vi "MOKE_Teperature and FIeld Sweep_1022D.vi"() -> ()   [LabVIEW 2022 SP3]
uses:
  <vilib>/Analysis/baseanly.llb/Mean (DBL).vi
  <vilib>/Utility/file.llb/Write Delimited Spreadsheet (string).vi
  <vilib>/Utility/file.llb/Write Delimited Spreadsheet (DBL).vi
  <vilib>/Analysis/NI_AALBase.lvlib
panel:
  in  "Num Averages":i32=100
  in  "Read Status":bool
  in  "Wait for position/focus check every (Oe)":i32
  out "Rh1 B/A v F":cluster{dbl[], dbl[]}(graph)
  out "Temperature Status":i32(ring) items=["TemperatureUnknown"=0, "Stable"=1, "Tracking"=2, "Near"=5, "Chasing"=6, "Filling"=7, "Standby"=10, "Disabled"=13, "ImpedanceNotFunction"=14, "TempFailure"=15]
  out "Field Status":i32(ring) items=["MagnetUnknown"=0, "StablePersistent"=1, "WarmingSwitch"=2, "CoolingSwitch"=3, "StableDriven"=4, "Iterating"=5, "Charging"=6, "Discharging"=7, "CurrentError"=8, "MagnetFailure"=15]
  out "Field":dbl
  out "Temperature":dbl
  in  "Initialize":bool
  in  "System Stablization (s)":dbl=0.1 format="%#_13g"
  in  "Low Value (Oe)":dbl=-30000.0
  in  "High Value (Oe)":dbl=30000.0
  in  "Sweep Field Approach":i32(ring) items=["Linear", "NoOvershoot", "Oscillate"]
  in  "Sweep F Rate (Oe/s)":dbl=200.0 format="%#_13g"
  in  "Sweep F mode":i32(ring) items=["Persistent", "Driven"]
  in  "Set Fixed T":dbl=2.0
  in  "Fixed Temperature Approach":i32(ring)=1 items=["FastSettle", "NoOvershoot"]
  in  "FIxed T  Rate (K/min)":dbl=20.0
  out "PhaseA-F":cluster{dbl[], dbl[]}(graph)
  out "RA-F":cluster{dbl[], dbl[]}(graph)
  out "Phaseh1B-F":cluster{dbl[], dbl[]}(graph)
  out "Rh1B-F":cluster{dbl[], dbl[]}(graph)
  out "phase B 2":dbl
  in  "Phase B 2":u16(ring)=3 items=["X", "Y", "R", "Theta", "Frequency", "Noise", "Xh1", "Yh1", "Rh1", "Theta h1", "Xh2", "Yh2", "Rh2", "Theta h2"]
  out "phase A 2":dbl
  in  "Phase A 2":u16(ring)=3 items=["X", "Y", "R", "Theta", "Frequency", "Noise", "Xh1", "Yh1", "Rh1", "Theta h1", "Xh2", "Yh2", "Rh2", "Theta h2"]
  out "para1 Measurement (mV) 2":dbl=1.49013e-07
  in  "F Clear Plot A":bool
  in  "Parameter A 2":u16(ring)=2 items=["X", "Y", "R", "Theta", "Frequency", "Noise", "Xh1", "Yh1", "Rh1", "Theta h1", "Xh2", "Yh2", "Rh2", "Theta h2"]
  out "para2 Measurement (uV) 2":dbl=1.49013e-07
  in  "F Clear Plot B":bool
  in  "Parameter B 2":u16(ring)=2 items=["X", "Y", "R", "Theta", "Frequency", "Noise", "Xh1", "Yh1", "Rh1", "Theta h1", "Xh2", "Yh2", "Rh2", "Theta h2"]
  out "Field Setting":dbl format="%#_13g"
  out "Fixed Temperature":dbl
  out "Measured Field":dbl
  out "Field Status":i32(ring) items=["MagnetUnknown"=0, "StablePersistent"=1, "WarmingSwitch"=2, "CoolingSwitch"=3, "StableDriven"=4, "Iterating"=5, "Charging"=6, "Discharging"=7, "CurrentError"=8, "MagnetFailure"=15]
  out "Temperature Status":i32(ring) items=["TemperatureUnknown"=0, "Stable"=1, "Tracking"=2, "Near"=5, "Chasing"=6, "Filling"=7, "Standby"=10, "Disabled"=13, "ImpedanceNotFunction"=14, "TempFailure"=15]
  out "Measuring F":bool
  in  "Step(Oe)":i32=2000
  out "F loop run":i32
  out "Temperature Status":i32(ring) items=["TemperatureUnknown"=0, "Stable"=1, "Tracking"=2, "Near"=5, "Chasing"=6, "Filling"=7, "Standby"=10, "Disabled"=13, "ImpedanceNotFunction"=14, "TempFailure"=15]
  out "Field Status":i32(ring) items=["MagnetUnknown"=0, "StablePersistent"=1, "WarmingSwitch"=2, "CoolingSwitch"=3, "StableDriven"=4, "Iterating"=5, "Charging"=6, "Discharging"=7, "CurrentError"=8, "MagnetFailure"=15]
  out "Fixed Field":dbl
  out "Measured Temperature":dbl
  in  "Delay(T/F)":dbl=5.0
  in  "Set FIxed F (Oe)":dbl format="%#_13g"
  in  "Fixed Field Approach":i32(ring) items=["Linear", "NoOvershoot", "Oscillate"]
  in  "FIxed F Rate (Oe/s)":dbl=100.0 format="%#_13g"
  in  "Fixed F mode":i32(ring) items=["Persistent", "Driven"]
  in  "Sweep Temperature Approach":i32(ring)=1 items=["FastSettle", "NoOvershoot"]
  in  "Sweep T  Rate (K/min)":dbl=10.0
  in  "Sweep T/F":bool
  in  "Remote":bool=TRUE
  in  "IP Address":string="169.254.170.239"
  out "Measuring T":bool
  in  "A Sine Output Amplitude (V)":sgl=0.1
  in  "path (folder + filename)":string="C:\\Users\\Public\\OneDrive\\Desktop\\MOKE program\\sweep files"
  in  "LOCKIN address":refnum<visa-resource-name>="COM3"
  out "PhaseA-T":cluster{dbl[], dbl[]}(graph)
  out "RA-T":cluster{dbl[], dbl[]}(graph)
  out "Phaseh1-T":cluster{dbl[], dbl[]}(graph)
  out "Rh1B-T":cluster{dbl[], dbl[]}(graph)
  out "phase B":dbl
  in  "Phase B":u16(ring)=9 items=["X", "Y", "R", "Theta", "Frequency", "Noise", "Xh1", "Yh1", "Rh1", "Theta h1", "Xh2", "Yh2", "Rh2", "Theta h2"]
  out "phase A":dbl
  in  "Phase A":u16(ring)=3 items=["X", "Y", "R", "Theta", "Frequency", "Noise", "Xh1", "Yh1", "Rh1", "Theta h1", "Xh2", "Yh2", "Rh2", "Theta h2"]
  out "para1 Measurement (mV)":dbl=1.49013e-07
  in  "T Clear Plot A":bool
  in  "Parameter A":u16(ring)=2 items=["X", "Y", "R", "Theta", "Frequency", "Noise", "Xh1", "Yh1", "Rh1", "Theta h1", "Xh2", "Yh2", "Rh2", "Theta h2"]
  out "para2 Measurement (uV)":dbl=1.49013e-07
  in  "T Clear Plot B":bool
  in  "Parameter B":u16(ring)=8 items=["X", "Y", "R", "Theta", "Frequency", "Noise", "Xh1", "Yh1", "Rh1", "Theta h1", "Xh2", "Yh2", "Rh2", "Theta h2"]
  out "Temperature Setting":dbl format="%#_13g"
  in  "Save data or not":bool=TRUE
  in  "Step(K)":i32=10
  out "T loop run":i32
  in  "B frequency":dbl=267.7 format="%#_13g"
  in  "B Input Connection (0: Single-Ended)":u16(ring)=1 items=["Single-Ended Voltage", "Differential Voltage", "1 MOhm Current Gain", "100 MOhm Current Gain"]
  in  "B harmonic 1":u8=2
  in  "B harmonic 2":u8=3
  in  "B reference Manual Phase":dbl=-59.75
  in  "auto phase B":bool=TRUE
  in  "B Sample time (s)":dbl=0.001 min=0.001 max=100.0 step=0.001
  in  "B Sensitivity":u16(ring)=20 items=["1 nV/fA", "2 nV/fA", "5 nV/fA", "10 nV/fA", "20 nV/fA", "50 nV/fA", "100 nV/fA", "200 nV/fA", "500 nV/fA", "1 uV/pA", "2 uV/pA", "5 uV/pA", "10 uV/pA", "20 uV/pA", "50 uV/pA", "100 uV/pA", "200 uV/pA", "500 uV/pA", "1 mV/nA", "2 mV/nA", "5 mV/nA", "10 mV/nA", "20 mV/nA", "50 mV/nA", "100 mV/nA", "200 mV/nA", "500 mV/nA", "1 V/uA"]
  in  "Enable Sync Filter B (open when f<200Hz)":bool
  in  "B Time Constant":u8(ring)=9 items=["10 us", "30 us", "100 us", "300 us", "1 ms", "3 ms", "10 ms", "30 ms", "100 ms", "300 ms", "1 s", "3 s", "10 s", "30 s", "100 s", "300 s", "1 ks", "3 ks"]
  in  "B Reference Source":u8(ring) items=["External", "Internal", "Internal Sweep", "Channel-A"]
  in  "B Low Pass Filter Slope":u8(ring)=2 items=["6 dB/oct", "12 dB/oct", "18 db/oct", "24 dB/oct"]
  in  "A frequency":dbl=267.7 format="%#_13g"
  in  "A Input Connection (0: Single-Ended)":u16(ring)=1 items=["Single-Ended Voltage", "Differential Voltage", "1 MOhm Current Gain", "100 MOhm Current Gain"]
  in  "A harmonic 1":u8=2
  in  "A harmonic 2":u8=3
  in  "A reference Manual Phase":dbl=-59.75
  in  "auto phase A":bool=TRUE
  in  "A Reference Source":u8(ring)=1 items=["External", "Internal", "Internal Sweep"]
  in  "A Sample time (s)":dbl=0.001 min=0.001 max=100.0 step=0.001
  in  "A Time Constant":u8(ring)=9 items=["10 us", "30 us", "100 us", "300 us", "1 ms", "3 ms", "10 ms", "30 ms", "100 ms", "300 ms", "1 s", "3 s", "10 s", "30 s", "100 s", "300 s", "1 ks", "3 ks"]
  in  "Enable Sync Filter A (open when f<200Hz)":bool
  in  "A Sensitivity":u16(ring)=20 items=["1 nV/fA", "2 nV/fA", "5 nV/fA", "10 nV/fA", "20 nV/fA", "50 nV/fA", "100 nV/fA", "200 nV/fA", "500 nV/fA", "1 uV/pA", "2 uV/pA", "5 uV/pA", "10 uV/pA", "20 uV/pA", "50 uV/pA", "100 uV/pA", "200 uV/pA", "500 uV/pA", "1 mV/nA", "2 mV/nA", "5 mV/nA", "10 mV/nA", "20 mV/nA", "50 mV/nA", "100 mV/nA", "200 mV/nA", "500 mV/nA", "1 V/uA"]
  in  "A Low Pass Filter Slope":u8(ring)=2 items=["6 dB/oct", "12 dB/oct", "18 db/oct", "24 dB/oct"]
  in  "stabilization(S)":dbl=0.1 format="%#_13g"
  in  "High Value (K)":dbl=300.0
  in  "Low Value (K)":dbl=2.0
  in  "loop #":i32=1
  # "Status"
  # "opticool ip addresse: 169.254.170.239"
  # "Lock-in Setting"
  # "Channel A"
  # "Channel B"
  # "Sweep F Mesurement"
  # "Temprature and Field Setting"
  # "Sweep T Mesurement"
  # "Sweep F"
  # "Sweep T"
  # "0 for no checks"
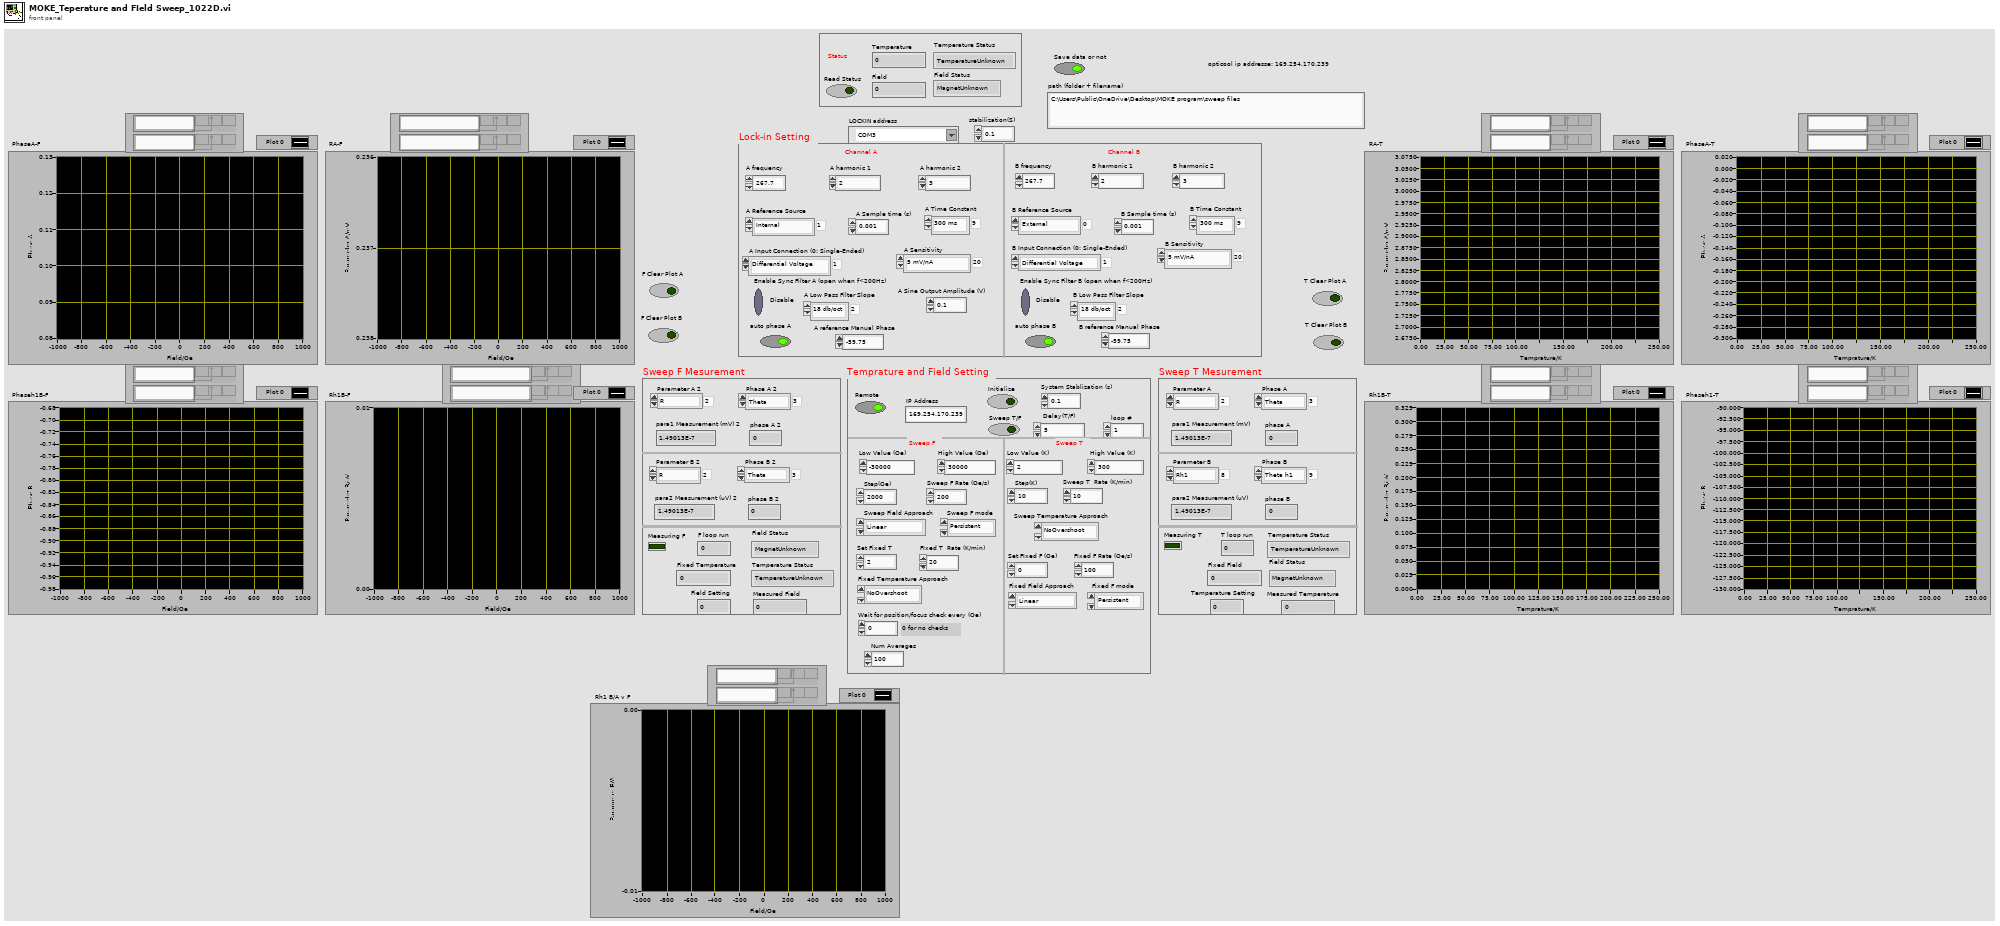
[diagram p1: front panel]
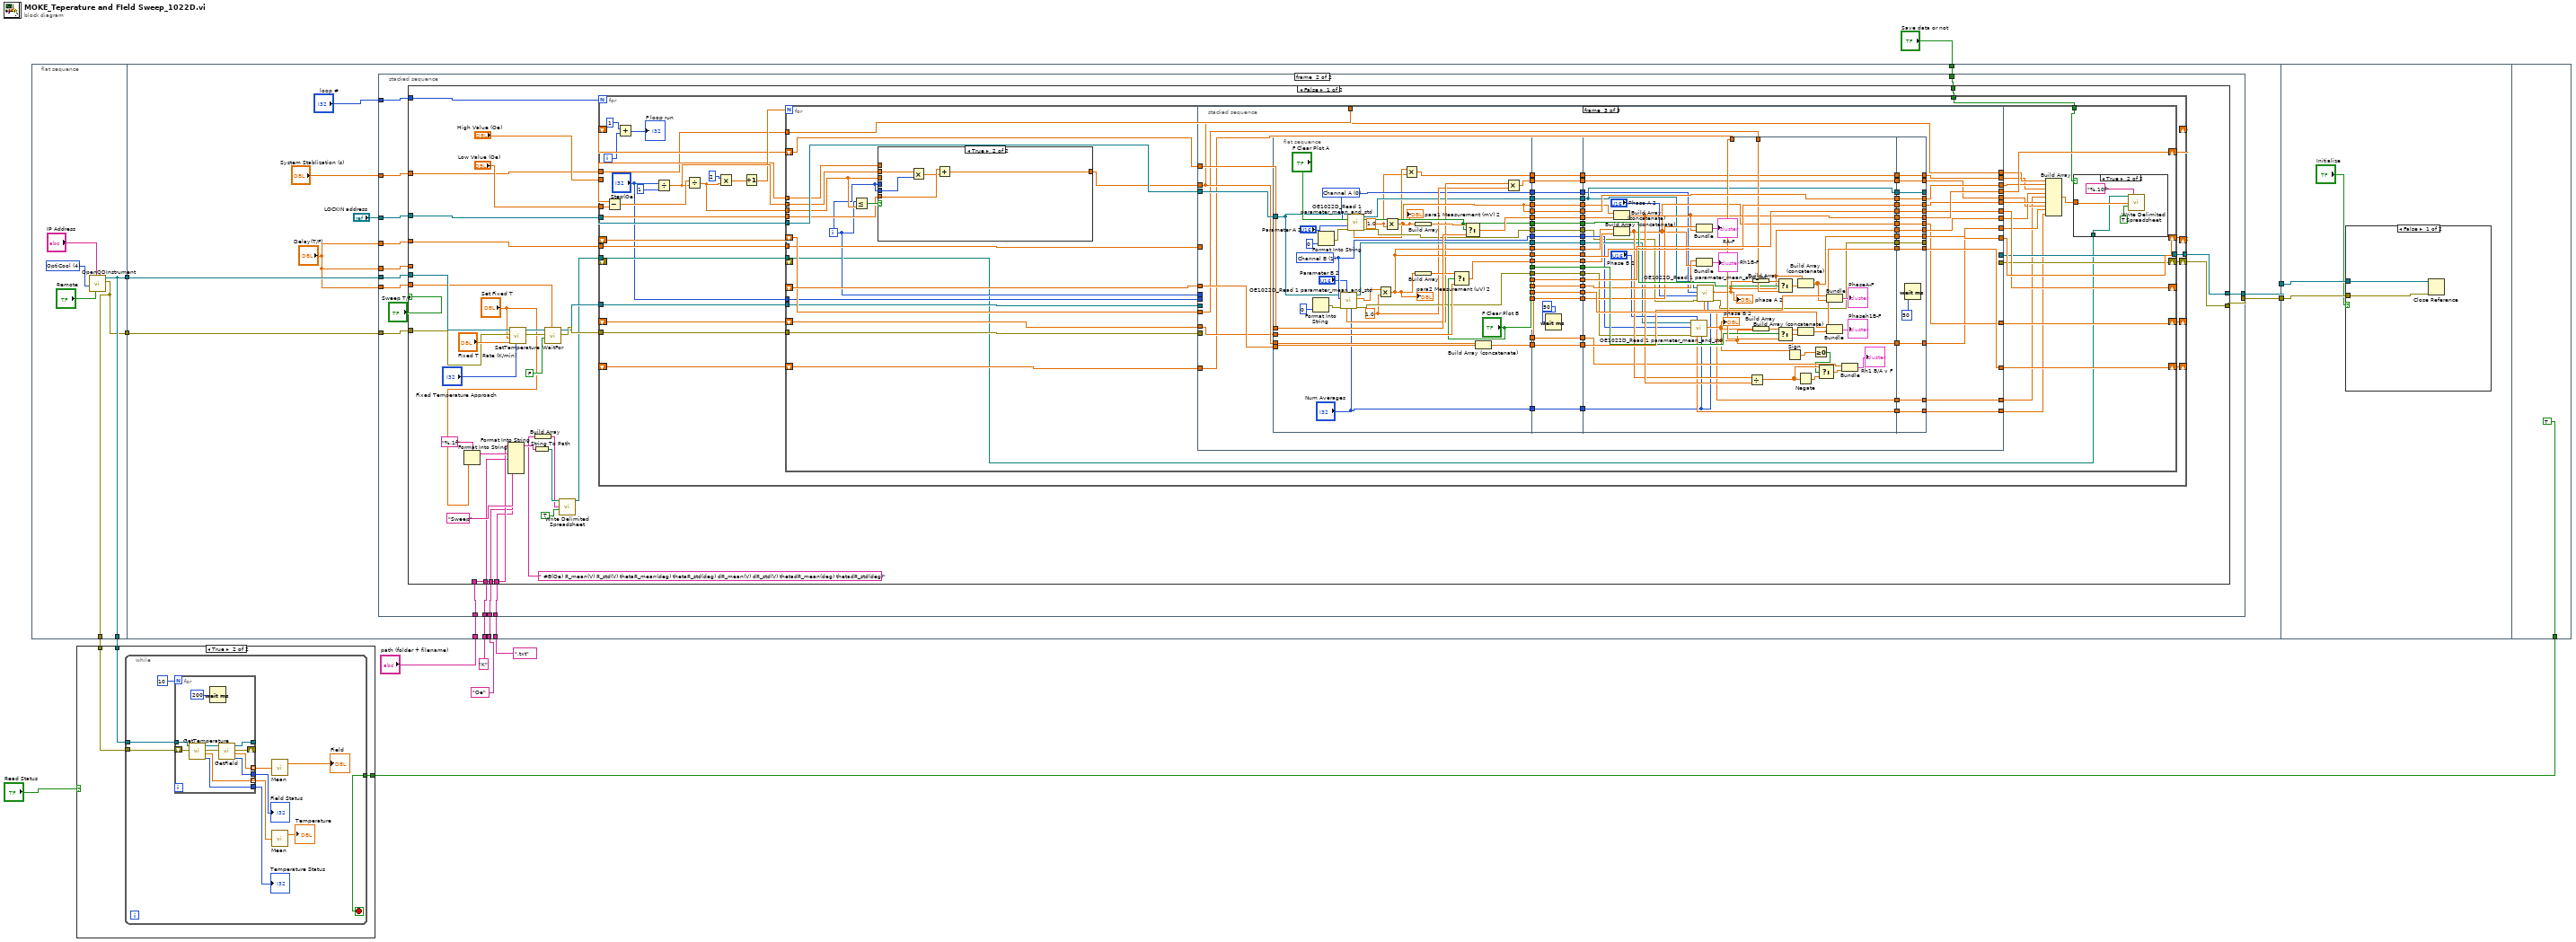
[diagram p0: block diagram]
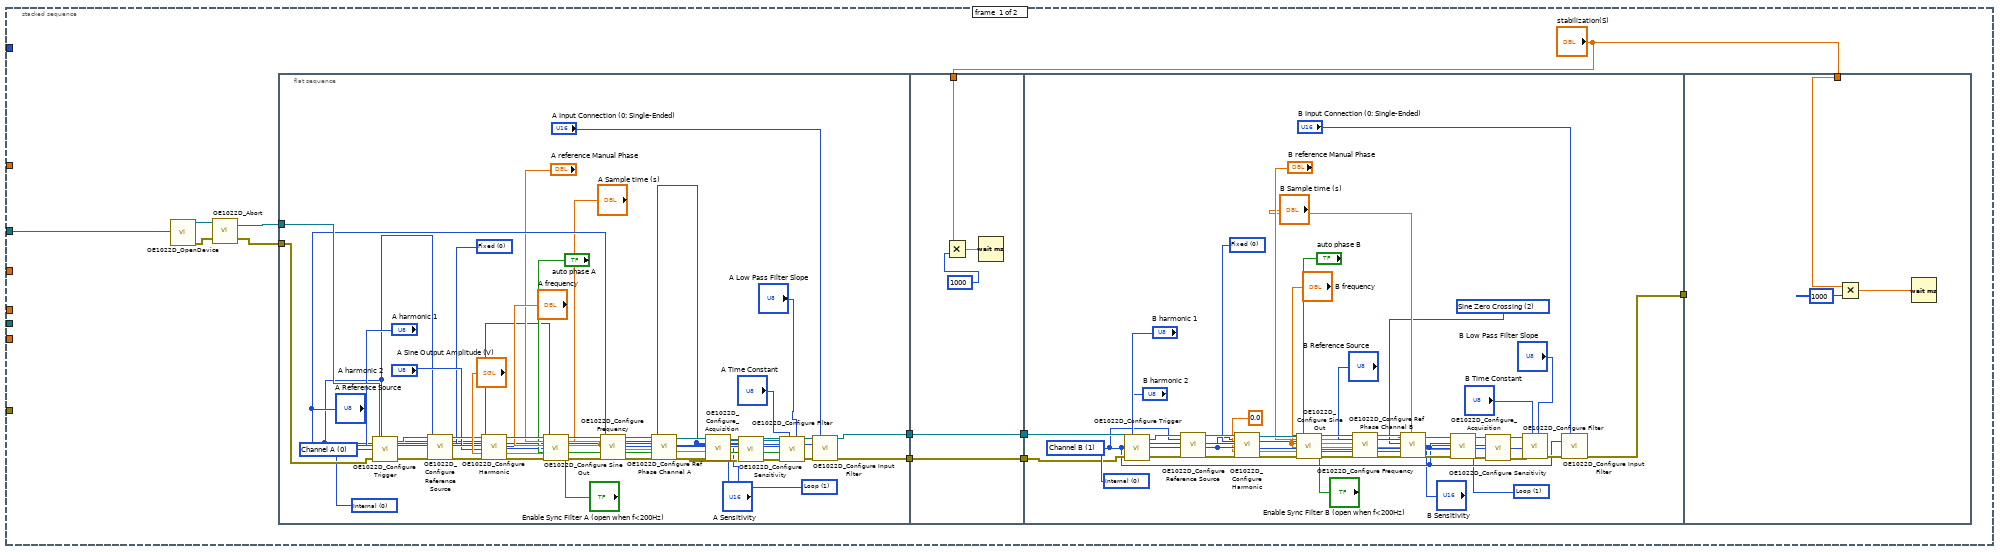
[diagram p3: hidden frame]
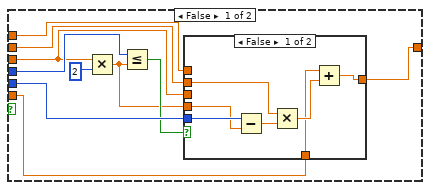
[diagram p5: hidden frame]
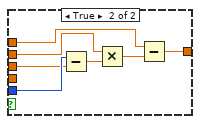
[diagram p6: hidden frame]
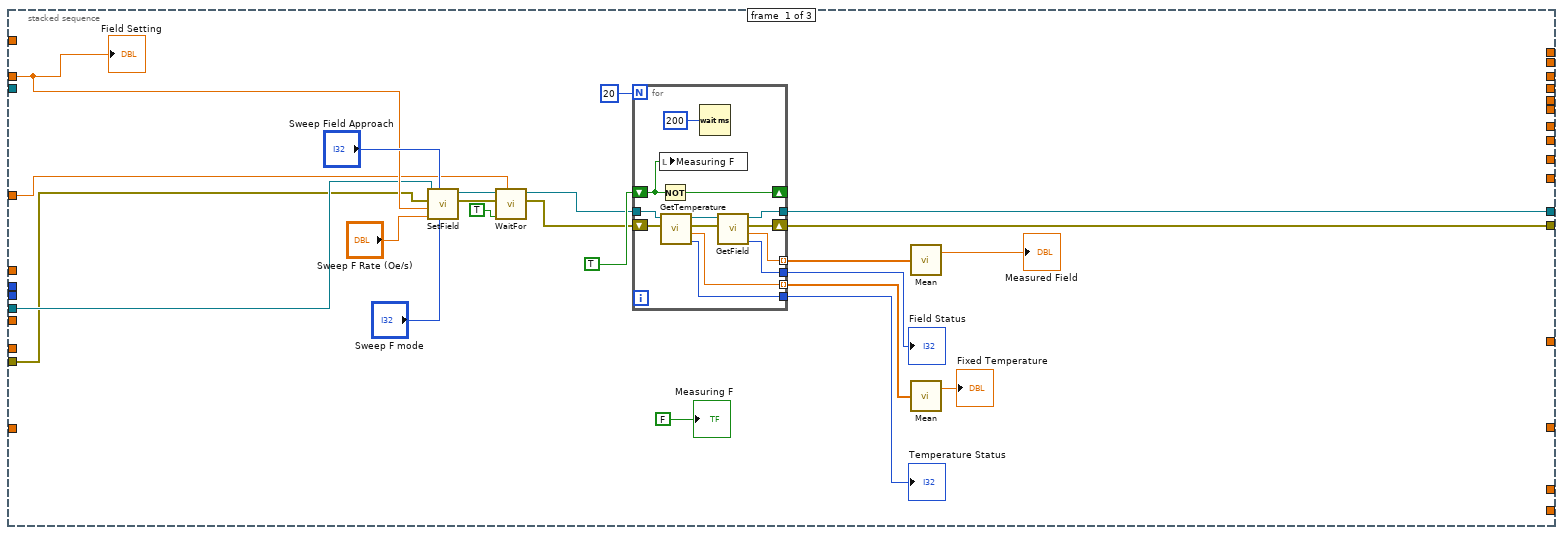
[diagram p7: hidden frame]
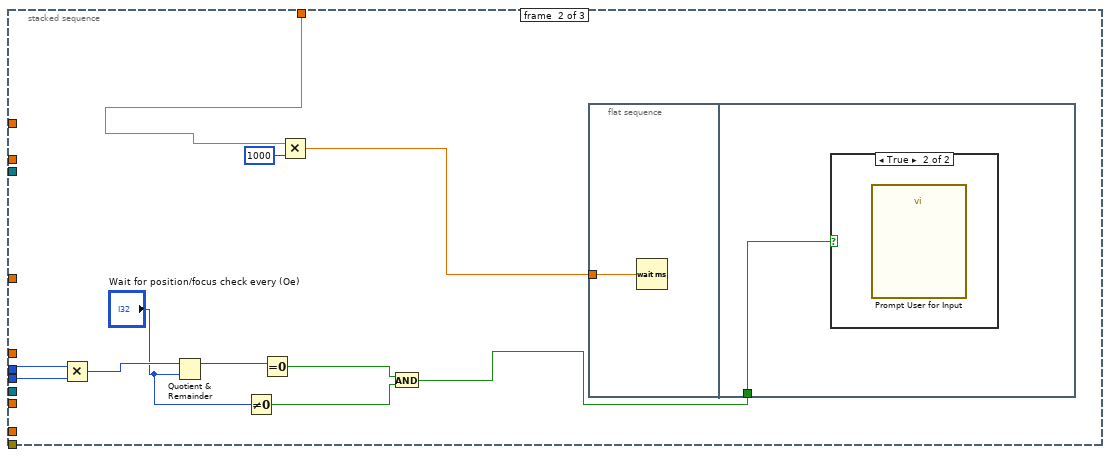
[diagram p8: hidden frame]
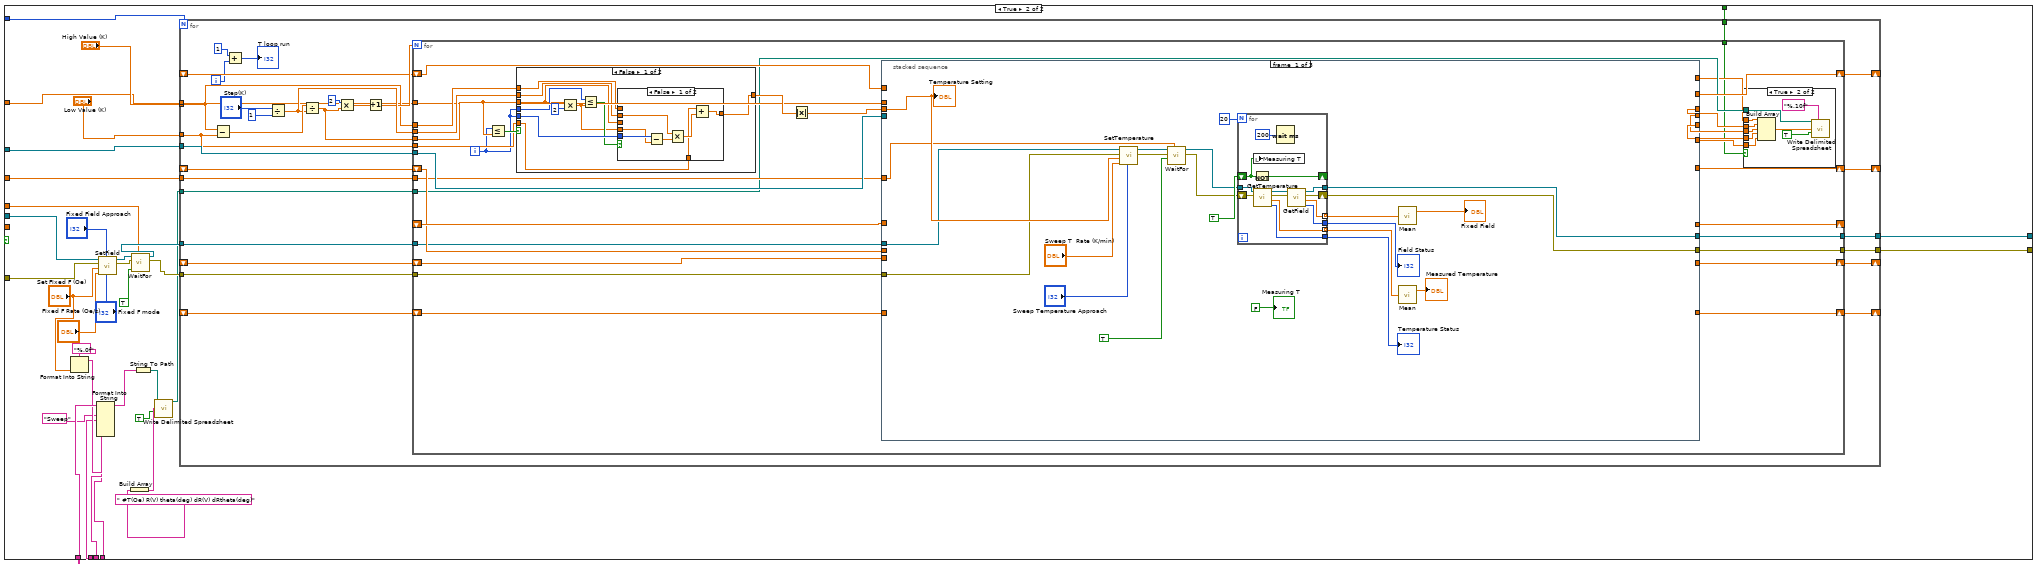
[diagram p10: hidden frame]
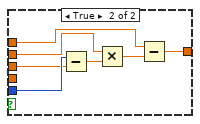
[diagram p12: hidden frame]
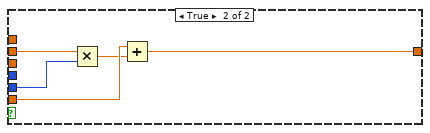
[diagram p13: hidden frame]
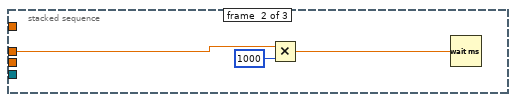
[diagram p14: hidden frame]
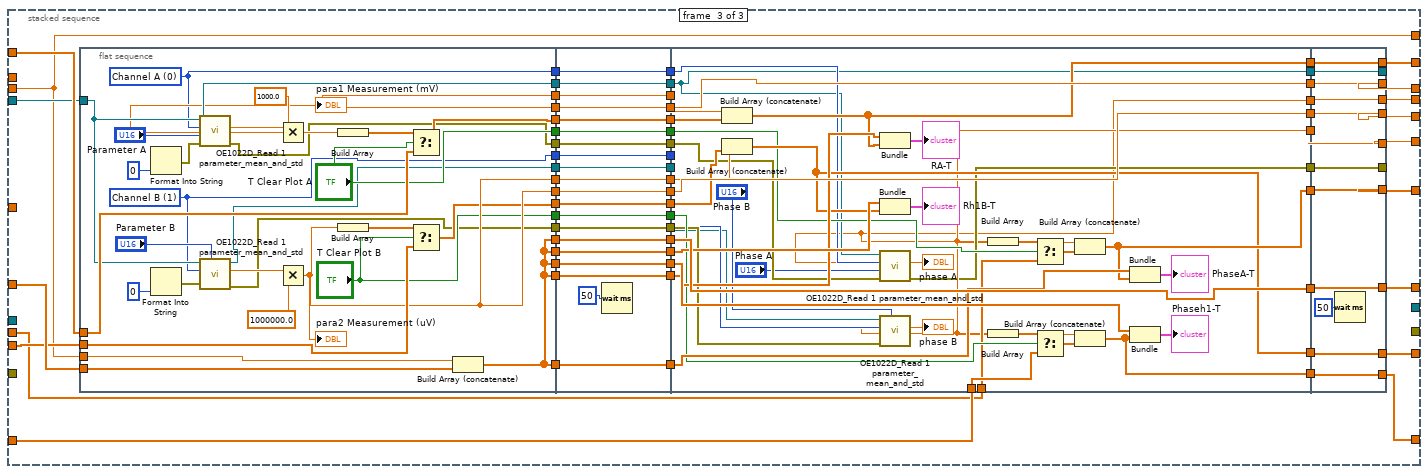
[diagram p15: hidden frame]
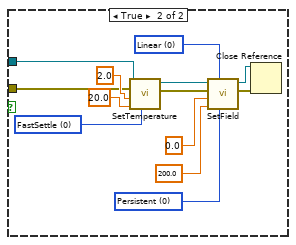
[diagram p16: hidden frame]
diagram:
  n1 = flat-sequence {
    tunnel: [w15] -> w13
    tunnel: [w14] -> w12
    tunnel: [w15] -> w5
    tunnel: [w14] -> w4
    tunnel: w13 -> [w29]
    tunnel: w12 -> [w28]
    tunnel: "path (folder + filename)" -> [w26]
    tunnel: "Oe" -> [w25]
    tunnel: "K" -> [w24]
    tunnel: ".txt" -> [w23]
    tunnel: [w21] -> w7
    tunnel: [w20] -> w6
    tunnel: "Save data or not" -> [w19]
    tunnel: w7 -> [w871]
    tunnel: w6 -> [w870]
    tunnel: [TRUE] -> w2
    frame #0 {
      w16 = 4 items=["PPMS", "VersaLab", "DynaCool", "SVSM", "OptiCool"] ("InstrumentType")
      n2 = call "OpenQDInstrument.vi"("Remote"="Remote", "IP Address"="IP Address", "InstrumentType"=w16) -> ("error out"=w14:errorcluster, "Instrument Ref"=w15:refnum<k24>)  [unwired: 5 in]
    }
    frame #1 {
      n3 = stacked-sequence {
        tunnel: "LOCKIN address" -> [w34 w143]
        tunnel: "loop #" -> [_ w142]
        tunnel: w29 -> [_ w140]
        tunnel: w28 -> [_ w139]
        tunnel: "Delay(T/F)" -> [_ w138]
        tunnel: "Delay(T/F)" -> [_ w137]
        tunnel: "Delay(T/F)" -> [_ w136]
        tunnel: w26 -> [_ w135]
        tunnel: w25 -> [_ w134]
        tunnel: w24 -> [_ w133]
        tunnel: w23 -> [_ w132]
        tunnel: "System Stablization (s)" -> [_ w131]
        tunnel: [_ w130] -> w21
        tunnel: [_ w129] -> w20
        tunnel: w19 -> [_ w128]
        frame #0 {
          n4 = call "OE1022D_OpenDevice.vi"("VISA resource name"=w34) -> ("VISA资源名称输出"=w33:refnum<visa-resource-name>, "错误输出"=w35:errorcluster)  [unwired: 17 in]
          n5 = call "OE1022D_Abort.vi"("error in (no error)"=w35, "VISA resource name"=w33) -> ("error out"=w40:errorcluster, "VISA resource name out"=w41:refnum<visa-resource-name>)
          n6 = flat-sequence {
            tunnel: w41 -> [w81]
            tunnel: [w69] -> w39
            tunnel: w40 -> [w80]
            tunnel: [w57] -> w37
            tunnel: w39 -> [w86]
            tunnel: [w86] -> w38
            tunnel: w37 -> [w85]
            tunnel: [w85] -> w36
            tunnel: "stabilization(S)" -> [w82]
            tunnel: w38 -> [w107]
            tunnel: [w106] -> w42
            tunnel: w36 -> [w105]
            tunnel: w42 -> [_]
            tunnel: "stabilization(S)" -> [w125]
            frame #0 {
              w43 = u8 1 items=["Single", "Loop"] ("Sample Mode (Single/Loop)")
              w56 = u8 0 items=["Fixed", "Linear", "Log"] ("SineOut Mode")
              w58 = u16 0 items=["Internal", "External"] ("Trigger Source (0: Internal)")
              w47 = u8 0 items=["Channel A", "Channel B"] ("OE1022D A/B")
              n7 = call "OE1022D_Configure Trigger.vi"("Trigger Source (0: Internal)"=w58, "error in (no error)   2"=w80, "OE1022D A/B"=w47, "VISA resource name   2"=w81) -> ("error out   2"=w74:errorcluster, "VISA resource name out   2"=w75:refnum<visa-resource-name>)
              n8 = call "OE1022D_Configure Reference Source.vi"("VISA resource name"=w75, "OE1022D A/B"=w47, "Reference Source"="A Reference Source", "error in (no error)"=w74) -> ("VISA resource name out"=w73:refnum<visa-resource-name>, "error out"=w71:errorcluster)  [unwired: 14 in]
              n9 = call "OE1022D_Configure Harmonic.vi"("VISA resource name"=w73, "OE1022D A/B"=w47, "Harmonic 1"="A harmonic 1", "Harmonic 2"="A harmonic 2", "error in (no error)"=w71) -> ("VISA resource name out"=w72:refnum<visa-resource-name>, "error out"=w70:errorcluster)  [unwired: 13 in]
              n10 = call "OE1022D_Configure Sine Out.vi"("VISA resource name"=w72, "SineOut Mode"=w56, "OE1022D A/B"=w47, "Sine Output Amplitude (V)"="A Sine Output Amplitude (V)", "error in (no error)"=w70) -> ("VISA resource name out"=w78:refnum<visa-resource-name>, "error out"=w77:errorcluster)  [unwired: 9 in]
              n11 = call "OE1022D_Configure Frequency.vi"("VISA resource name"=w78, "OE1022D A/B"=w47, "Internal Frequency(Hz)"="A frequency", "error in (no error)"=w77) -> ("VISA resource name out"=w68:refnum<visa-resource-name>, "error out"=w65:errorcluster)  [unwired: 14 in]
              n12 = call "OE1022D_Configure Ref Phase Channel A.vi"("VISA resource name"=w68, "Reference Source"="A Reference Source", "Internal Frequency(Hz)"="A frequency", "Auto Phase (T: Enabled)"="auto phase A", "error in (no error)"=w65, "Manual Phase  (degree)"="A reference Manual Phase") -> ("VISA resource name out"=w67:refnum<visa-resource-name>, "error out"=w66:errorcluster)  [unwired: 12 in]
              n13 = call "OE1022D_Configure_Acquisition.vi"("VISA resource name"=w67, "OE1022D A/B"=w47, "Sample time (s)"="A Sample time (s)", "error in (no error)"=w66, "Sample Mode (Single/Loop)"=w43) -> ("VISA resource name out"=w50:refnum<visa-resource-name>, "error out"=w49:errorcluster)  [unwired: 3 in]
              n14 = call "OE1022D_Configure Sensitivity.vi"("VISA resource name"=w50, "OE1022D A/B"=w47, "Sensitivity"="A Sensitivity", "error in (no error)"=w49) -> ("VISA resource name out"=w54:refnum<visa-resource-name>, "error out"=w53:errorcluster)  [unwired: 14 in]
              n15 = call "OE1022D_Configure Filter.vi"("Low Pass Filter Slope (1: 12dB/oct)"="A Low Pass Filter Slope", "Time Constant (8: 100ms)"="A Time Constant", "error in (no error)"=w53, "Enable Sync Filter (F: Disable)"="Enable Sync Filter A (open when f<200Hz)", "OE1022D A/B"=w47, "VISA resource name"=w54) -> ("error out"=w51:errorcluster, "VISA resource name out"=w52:refnum<visa-resource-name>)  [unwired: 4 in]
              n16 = call "OE1022D_Configure Input Filter.vi"("VISA resource name"=w52, "Input Source"="A Input Connection (0: Single-Ended)", "OE1022D A/B"=w47, "error in (no error)"=w51) -> ("VISA resource name out"=w57:refnum<visa-resource-name>, "error out"=w69:errorcluster)  [unwired: 10 in]
            }
            frame #1 {
              n17 = Multiply(x=w82, y=1000) -> (x*y=w84:dbl)
              n18 = Wait (ms)(milliseconds to wait=w84) -> ()  [unwired: 1 out]
            }
            frame #2 {
              w87 = u8 1 items=["Single", "Loop"] ("Sample Mode (Single/Loop)")
              w89 = u8 2 items=["TTL Pos", "TTL Neg", "Sine Zero Crossing"] ("External Ref Trigger")
              w102 = u8 0 items=["Fixed", "Linear", "Log"] ("SineOut Mode")
              w108 = u16 0 items=["Internal", "External"] ("Trigger Source (0: Internal)")
              w94 = u8 1 items=["Channel A", "Channel B"] ("OE1022D A/B")
              n19 = call "OE1022D_Configure Trigger.vi"("Trigger Source (0: Internal)"=w108, "error in (no error)   2"=w107, "OE1022D A/B"=w94, "VISA resource name   2"=w105) -> ("error out   2"=w120:errorcluster, "VISA resource name out   2"=w121:refnum<visa-resource-name>)
              n20 = call "OE1022D_Configure Reference Source.vi"("VISA resource name"=w121, "OE1022D A/B"=w94, "error in (no error)"=w120) -> ("VISA resource name out"=w119:refnum<visa-resource-name>, "error out"=w117:errorcluster)  [unwired: 15 in]
              n21 = call "OE1022D_Configure Harmonic.vi"("VISA resource name"=w119, "OE1022D A/B"=w94, "Harmonic 1"="B harmonic 1", "Harmonic 2"="B harmonic 2", "error in (no error)"=w117) -> ("VISA resource name out"=w118:refnum<visa-resource-name>, "error out"=w116:errorcluster)  [unwired: 13 in]
              n22 = call "OE1022D_Configure Sine Out.vi"("VISA resource name"=w118, "SineOut Mode"=w102, "OE1022D A/B"=w94, "Sine Output Amplitude (V)"=sgl 0.0, "error in (no error)"=w116) -> ("VISA resource name out"=w123:refnum<visa-resource-name>, "error out"=w122:errorcluster)  [unwired: 9 in]
              n23 = call "OE1022D_Configure Frequency.vi"("VISA resource name"=w123, "OE1022D A/B"=w94, "Internal Frequency(Hz)"="B frequency", "error in (no error)"=w122) -> ("VISA resource name out"=w115:refnum<visa-resource-name>, "error out"=w112:errorcluster)  [unwired: 14 in]
              n24 = call "OE1022D_Configure Ref Phase Channel B.vi"("VISA resource name"=w115, "Reference Source"="B Reference Source", "External Ref Trigger"=w89, "Internal Frequency(Hz)"="B frequency", "Auto Phase (T: Enabled)"="auto phase B", "error in (no error)"=w112, "Manual Phase  (degree)"="B reference Manual Phase") -> ("VISA resource name out"=w114:refnum<visa-resource-name>, "error out"=w113:errorcluster)  [unwired: 11 in]
              n25 = call "OE1022D_Configure_Acquisition.vi"("VISA resource name"=w114, "OE1022D A/B"=w94, "Sample time (s)"="B Sample time (s)", "error in (no error)"=w113, "Sample Mode (Single/Loop)"=w87) -> ("VISA resource name out"=w95:refnum<visa-resource-name>, "error out"=w96:errorcluster)  [unwired: 3 in]
              n26 = call "OE1022D_Configure Sensitivity.vi"("VISA resource name"=w95, "OE1022D A/B"=w94, "Sensitivity"="B Sensitivity", "error in (no error)"=w96) -> ("VISA resource name out"=w99:refnum<visa-resource-name>, "error out"=w98:errorcluster)  [unwired: 14 in]
              n27 = call "OE1022D_Configure Filter.vi"("Low Pass Filter Slope (1: 12dB/oct)"="B Low Pass Filter Slope", "Time Constant (8: 100ms)"="B Time Constant", "error in (no error)"=w98, "Enable Sync Filter (F: Disable)"="Enable Sync Filter B (open when f<200Hz)", "OE1022D A/B"=w94, "VISA resource name"=w99) -> ("error out"=w97:errorcluster)  [unwired: 4 in, 1 out]
              n28 = call "OE1022D_Configure Input Filter.vi"("Input Source"="B Input Connection (0: Single-Ended)", "OE1022D A/B"=w94, "error in (no error)"=w97) -> ("error out"=w106:errorcluster)  [unwired: 11 in, 1 out]
            }
            frame #3 {
              n29 = Multiply(x=w125, y=1000) -> (x*y=w127:dbl)
              n30 = Wait (ms)(milliseconds to wait=w127) -> ()  [unwired: 1 out]
            }
          }
        }
        frame #1 {
          n31 = case shown="False" "Sweep T/F" {
            tunnel: w143 -> [w175 w565]
            tunnel: w142 -> [w176 w564]
            tunnel: w140 -> [w167 w560]
            tunnel: w139 -> [w168 w559]
            tunnel: w138 -> [_ w553]
            tunnel: w137 -> [w174 w552]
            tunnel: w136 -> [w166 _]
            tunnel: w135 -> [w158 w548]
            tunnel: w134 -> [w157 w544]
            tunnel: w133 -> [w156 w545]
            tunnel: w132 -> [w155 w543]
            tunnel: w131 -> [w152 w540]
            tunnel: [w151 w539] -> w130
            tunnel: [w150 w538] -> w129
            tunnel: w128 -> [w149 w537]
            frame False {
              n32 = Format Into String(format string="%.1f", "Set Fixed T") -> (resulting string=w160:string)  [unwired: 2 in, 1 out]
              n33 = Format Into String(initial string=w158, w160, w156, "Sweep", w157, w155) -> (resulting string=w161:string)  [unwired: 2 in, 1 out]
              n34 = call "SetTemperature.vi"("Approach"="Fixed Temperature Approach", "Rate"="FIxed T  Rate (K/min)", "Temperature"="Set Fixed T", "error in (no error)"=w168, "Instrument Ref In"=w167) -> ("error out"=w169:errorcluster, "Instrument Ref Out"=w170:refnum<k24>)  [unwired: 2 in, 1 out]
              n35 = String To Path(string=w161) -> (path=w148:path)
              n36 = Build Array(" #B(Oe) R_mean(V) R_std(V) thetaR_mean(deg) thetaR_std(deg) dR_mean(V) dR_std(V) thetadR_mean(deg) thetadR_std(deg)") -> (w146:string[])
              n37 = call "WaitFor.vi"("Delay"=w166, "Wait For Temperature"=FALSE ("WaitForTemperature"), "error in (no error)"=w169, "Instrument Ref In"=w170) -> ("error out"=w165:errorcluster, "Instrument Ref Out"=w164:refnum<k24>)  [unwired: 6 in]
              n38 = call-poly <vilib>:"Write Delimited Spreadsheet.vi"("file path (dialog if empty)"=w148, "1D data"=w146, "append to file? (new file:F)"=TRUE) -> ("new file path (Not A Path if cancelled)"=w145:path)  [unwired: 11 in, 1 out]
              n39 = for {
                N: w176 -> [_]
                tunnel: w175 -> [w206]
                tunnel: "Low Value (Oe)" -> [w201]
                tunnel: "High Value (Oe)" -> [w191]
                tunnel: w145 -> [w200]
                shift-right: [w196] -> _
                shift-left: _ -> [w195]
                shift-right: [w190] -> _
                shift-left: _ -> [w189]
                shift-right: [w188] -> _
                shift-left: _ -> [w187]
                shift-right: [w186] -> _
                shift-left: _ -> [w185]
                tunnel: w164 -> [w184]
                tunnel: w165 -> [w183]
                tunnel: w174 -> [w182]
                tunnel: w152 -> [w181]
                shift-right: [w180] -> w151
                shift-left: _ -> [_]
                tunnel: [w179] -> w150
                tunnel: w149 -> [w178]
                i -> [w193]
                n40 = Subtract(x=w191, y=w201) -> (x-y=w203:dbl)
                n41 = Add(x=1, y=w193) -> (x+y=→"F loop run":i32)
                n42 = Divide(x="Step(Oe)", y=1) -> (x/y=w202:dbl)
                n43 = Divide(x=w203, y=w202) -> (x/y=w199:dbl)
                n44 = Multiply(x=2, y=w199) -> (x*y=w198:dbl)
                n45 = Increment(x=w198) -> (x+1=w197:dbl)
                n46 = for {
                  N: w197 -> [_]
                  tunnel: w206 -> [w243]
                  tunnel: w202 -> [w239]
                  shift-right: [w232] -> w196
                  shift-left: w195 -> [w242]
                  tunnel: w199 -> [w237]
                  tunnel: w201 -> [w240]
                  tunnel: w191 -> [w238]
                  tunnel: w200 -> [w217]
                  shift-right: [w231] -> _
                  shift-left: _ -> [w235]
                  shift-right: [w234] -> w190
                  shift-left: w189 -> [w233]
                  shift-right: [w230] -> w188
                  shift-left: w187 -> [w229]
                  shift-right: [w228] -> w186
                  shift-left: w185 -> [w227]
                  tunnel: w184 -> [w226]
                  tunnel: w183 -> [w225]
                  tunnel: w182 -> [w224]
                  tunnel: w181 -> [w223]
                  shift-right: [w222] -> w180
                  shift-left: _ -> [_]
                  tunnel: [w221] -> w179
                  tunnel: w178 -> [w220]
                  tunnel: "Step(Oe)" -> [w218]
                  i -> [w219]
                  n47 = Less Or Equal?(x=w219, y=w237) -> (x <= y?=w241:bool)
                  n48 = case shown="True" w241 {
                    tunnel: w240 -> [w248 w276]
                    tunnel: w219 -> [w257 w275]
                    tunnel: w239 -> [w256 w274]
                    tunnel: [w254 w272] -> w236
                    tunnel: w238 -> [w255 _]
                    tunnel: w237 -> [w250 _]
                    tunnel: w219 -> [w253 _]
                    frame False {
                      n49 = Multiply(x=w250, y=2) -> (x*y=w249:dbl)
                      n50 = Less Or Equal?(x=w253, y=w249) -> (x <= y?=w251:bool)
                      n51 = case shown="False" w251 {
                        tunnel: w257 -> [w264 w271]
                        tunnel: w256 -> [w262 w269]
                        tunnel: w255 -> [_ w267]
                        tunnel: [w260 w266] -> w254
                        tunnel: w250 -> [_ w265]
                        tunnel: w249 -> [w259 _]
                        tunnel: w248 -> [w258 _]
                        frame False {
                          n52 = Subtract(x=w264, y=w259) -> (x-y=w263:dbl)
                          n53 = Multiply(x=w262, y=w263) -> (x*y=w261:dbl)
                          n54 = Add(x=w258, y=w261) -> (x+y=w260:dbl)
                        }
                        frame True {
                          n55 = Subtract(x=w271, y=w265) -> (x-y=w270:dbl)
                          n56 = Multiply(x=w269, y=w270) -> (x*y=w268:dbl)
                          n57 = Subtract(x=w267, y=w268) -> (x-y=w266:dbl)
                        }
                      }
                    }
                    frame True {
                      n58 = Multiply(x=w274, y=w275) -> (x*y=w273:dbl)
                      n59 = Add(x=w276, y=w273) -> (x+y=w272:dbl)
                    }
                  }
                  n60 = stacked-sequence {
                    tunnel: w243 -> [_ _ w404]
                    tunnel: w236 -> [w282 _ w403]
                    tunnel: w242 -> [_ _ w406]
                    tunnel: [_ _ w405] -> w232
                    tunnel: [_ _ w391] -> w216
                    tunnel: [_ _ w403] -> w214
                    tunnel: [_ _ w402] -> w231
                    tunnel: w235 -> [_ _ w401]
                    tunnel: [_ _ w400] -> w211
                    tunnel: [_ _ w399] -> w234
                    tunnel: w233 -> [_ _ w392]
                    tunnel: [_ _ w398] -> w230
                    tunnel: w229 -> [_ _ w393]
                    tunnel: [_ _ w397] -> w228
                    tunnel: w227 -> [_ _ w396]
                    tunnel: [_ _ w395] -> w212
                    tunnel: [_ _ w394] -> w213
                    tunnel: w226 -> [w281 _ _]
                    tunnel: w225 -> [w280 _ _]
                    tunnel: w224 -> [w279 _ _]
                    tunnel: w223 -> [_ w321 _]
                    tunnel: [w278 _ _] -> w222
                    tunnel: [w277 _ _] -> w221
                    tunnel: w219 -> [_ w320 _]
                    tunnel: w218 -> [_ w319 _]
                    tunnel: [_ _ w336] -> w210
                    tunnel: [_ _ w332] -> w209
                    tunnel: [_ _ w330] -> w208
                    tunnel: [_ _ w328] -> w207
                    frame #0 {
                      n61 = call "SetField.vi"("Mode"="Sweep F mode", "Approach"="Sweep Field Approach", "Rate"="Sweep F Rate (Oe/s)", "Field"=w282, "error in (no error)"=w280, "Instrument Ref In"=w281) -> ("error out"=w286:errorcluster, "Instrument Ref Out"=w287:refnum<k24>)  [unwired: 1 in, 1 out]
                      n62 = call "WaitFor.vi"("Delay"=w279, "Wait For Field"=TRUE, "error in (no error)"=w286, "Instrument Ref In"=w287) -> ("error out"=w284:errorcluster, "Instrument Ref Out"=w283:refnum<k24>)  [unwired: 6 in]
                      n63 = for {
                        N: 20 -> [_]
                        shift-right: [w312] -> _
                        shift-left: TRUE -> [w310]
                        shift-right: [w307] -> w278
                        shift-left: w284 -> [w309]
                        tunnel: w283 -> [w306]
                        tunnel: [w304] -> w277
                        tunnel: [w301] -> w297
                        tunnel: [w300] -> w296
                        tunnel: [w302] -> w294 mode=indexing
                        tunnel: [w303] -> w295 mode=indexing
                        n64 = local write "Measuring F"(w310) -> ()
                        n65 = Not(x=w310) -> (.not. x?=w312:bool)
                        n66 = call "GetTemperature.vi"("error in (no error)"=w309, "Instrument Ref In"=w306) -> ("Temperature\nStatus"=w300:i32, "Temperature"=w303:dbl, "error out"=w308:errorcluster, "Instrument Ref Out"=w305:refnum<k24>)  [unwired: 3 in, 1 out]
                        n67 = Wait (ms)(milliseconds to wait=u32 200) -> ()  [unwired: 1 out]
                        n68 = call "GetField.vi"("error in (no error)"=w308, "Instrument Ref In"=w305) -> ("Field\nStatus"=w301:i32, "Field"=w302:dbl, "error out"=w307:errorcluster, "Instrument Ref Out"=w304:refnum<k24>)  [unwired: 3 in, 1 out]
                      }
                      "Field Status" <- w297
                      "Temperature Status" <- w296
                      n69 = call-poly <vilib>:"Mean.vi"("X"=w294) -> ("mean"=→"Measured Field":dbl)  [unwired: 1 out]
                      n70 = call-poly <vilib>:"Mean.vi"("X"=w295) -> ("mean"=→"Fixed Temperature":dbl)  [unwired: 1 out]
                      "Field Setting" <- w282
                      "Measuring F" <- FALSE
                    }
                    frame #1 {
                      n71 = Multiply(x=w320, y=w319) -> (x*y=w318:i32)
                      n72 = Quotient & Remainder(x=w318, y="Wait for position/focus check every (Oe)") -> (x-y*floor(x/y)=w317:i32)  [unwired: 1 out]
                      n73 = Not Equal To 0?(x="Wait for position/focus check every (Oe)") -> (x != 0?=w313:bool)
                      n74 = Equal To 0?(x=w317) -> (x = 0?=w316:bool)
                      n75 = Multiply(x=w321, y=1000) -> (x*y=w323:dbl)
                      n76 = And(x=w316, y=w313) -> (x .and. y?=w315:bool)
                      n77 = flat-sequence {
                        tunnel: w323 -> [w324]
                        tunnel: w315 -> [w325]
                        frame #0 {
                          n78 = Wait (ms)(milliseconds to wait=w324) -> ()  [unwired: 1 out]
                        }
                        frame #1 {
                          n79 = case shown="True" w325 {
                            frame False {
                            }
                            frame True {
                              n80 = call "Prompt User for Input"() -> ()  [unwired: 17 in, 3 out]
                            }
                          }
                        }
                      }
                    }
                    frame #2 {
                      n81 = flat-sequence {
                        tunnel: w406 -> [w439]
                        tunnel: w404 -> [w412]
                        tunnel: w403 -> [w438]
                        tunnel: w401 -> [w437]
                        tunnel: w396 -> [w434]
                        tunnel: [w417] -> w390
                        tunnel: [w427] -> w389
                        tunnel: [w429] -> w388
                        tunnel: [w428] -> w387
                        tunnel: [w429] -> w386
                        tunnel: [w429] -> w385
                        tunnel: [w429] -> w384
                        tunnel: [w429] -> w383
                        tunnel: [w427] -> w382
                        tunnel: [w433] -> w381
                        tunnel: [w428] -> w380
                        tunnel: [w432] -> w379
                        tunnel: ["F Clear Plot B"] -> w378
                        tunnel: ["F Clear Plot A"] -> w377
                        tunnel: [w422] -> w376
                        tunnel: [w425] -> w375
                        tunnel: [w421] -> w374
                        tunnel: [w416] -> w373
                        tunnel: [w413] -> w372
                        tunnel: [w429] -> w371
                        tunnel: [w409] -> w337
                        tunnel: [w408] -> w333
                        tunnel: ["Num Averages"] -> w326
                        tunnel: w390 -> [w465]
                        tunnel: [w465] -> w370
                        tunnel: w389 -> [w464]
                        tunnel: [w464] -> w369
                        tunnel: w388 -> [w463]
                        tunnel: [w463] -> w368
                        tunnel: w387 -> [w462]
                        tunnel: [w462] -> w367
                        tunnel: w386 -> [w461]
                        tunnel: [w461] -> w366
                        tunnel: w385 -> [w460]
                        tunnel: [w460] -> w365
                        tunnel: w384 -> [w459]
                        tunnel: [w459] -> w364
                        tunnel: w383 -> [w458]
                        tunnel: [w458] -> w363
                        tunnel: w382 -> [w457]
                        tunnel: [w457] -> w362
                        tunnel: w381 -> [w456]
                        tunnel: [w456] -> w361
                        tunnel: w380 -> [w455]
                        tunnel: [w455] -> w360
                        tunnel: w379 -> [w454]
                        tunnel: [w454] -> w359
                        tunnel: w378 -> [w453]
                        tunnel: [w453] -> w358
                        tunnel: w377 -> [w452]
                        tunnel: [w452] -> w357
                        tunnel: w376 -> [w451]
                        tunnel: [w451] -> w356
                        tunnel: w375 -> [w450]
                        tunnel: [w450] -> w355
                        tunnel: w374 -> [w449]
                        tunnel: [w449] -> w354
                        tunnel: w373 -> [w448]
                        tunnel: [w448] -> w353
                        tunnel: w372 -> [w447]
                        tunnel: [w447] -> w352
                        tunnel: [w445] -> w351
                        tunnel: w371 -> [w445]
                        tunnel: [w444] -> w338
                        tunnel: w337 -> [w444]
                        tunnel: [w443] -> w334
                        tunnel: w333 -> [w443]
                        tunnel: [w442] -> w327
                        tunnel: w326 -> [w442]
                        tunnel: w370 -> [w474]
                        tunnel: w369 -> [w515]
                        tunnel: w368 -> [w514]
                        tunnel: w367 -> [w513]
                        tunnel: w366 -> [w512]
                        tunnel: w365 -> [w492]
                        tunnel: w364 -> [w491]
                        tunnel: w363 -> [w508]
                        tunnel: w362 -> [w505]
                        tunnel: w361 -> [w504]
                        tunnel: w360 -> [w502]
                        tunnel: w359 -> [w501]
                        tunnel: w393 -> [w500]
                        tunnel: w358 -> [w499]
                        tunnel: w392 -> [w497]
                        tunnel: w357 -> [w496]
                        tunnel: w356 -> [w475]
                        tunnel: w355 -> [w476]
                        tunnel: w354 -> [w477]
                        tunnel: w353 -> [w471]
                        tunnel: w352 -> [w473]
                        tunnel: [w474] -> w350
                        tunnel: [w490] -> w349
                        tunnel: [w515] -> w348
                        tunnel: [w514] -> w347
                        tunnel: [w469] -> w346
                        tunnel: [w470] -> w345
                        tunnel: [w506] -> w344
                        tunnel: [w503] -> w343
                        tunnel: [w489] -> w342
                        tunnel: [w513] -> w341
                        tunnel: [w479] -> w340
                        tunnel: w351 -> [w488]
                        tunnel: [w481] -> w339
                        tunnel: w338 -> [w481]
                        tunnel: [w480] -> w335
                        tunnel: w334 -> [w480]
                        tunnel: [w468] -> w331
                        tunnel: [w467] -> w329
                        tunnel: w327 -> [w466]
                        tunnel: [w521] -> w394
                        tunnel: [w522] -> w395
                        tunnel: [w523] -> w397
                        tunnel: [w524] -> w398
                        tunnel: [w525] -> w399
                        tunnel: [w526] -> _
                        tunnel: [w527] -> w400
                        tunnel: [w528] -> w402
                        tunnel: [w529] -> w391
                        tunnel: [w530] -> w405
                        tunnel: [w531] -> _
                        tunnel: w350 -> [w531]
                        tunnel: w349 -> [w530]
                        tunnel: w348 -> [w529]
                        tunnel: w347 -> [w528]
                        tunnel: w346 -> [w527]
                        tunnel: w345 -> [w526]
                        tunnel: w344 -> [w525]
                        tunnel: w343 -> [w524]
                        tunnel: w342 -> [w523]
                        tunnel: w341 -> [w522]
                        tunnel: w340 -> [w521]
                        tunnel: [w519] -> w336
                        tunnel: w339 -> [w519]
                        tunnel: [w518] -> w332
                        tunnel: w335 -> [w518]
                        tunnel: [w517] -> w330
                        tunnel: w331 -> [w517]
                        tunnel: w329 -> [w516]
                        tunnel: [w516] -> w328
                        frame #0 {
                          w410 = 1.0 ("y")
                          w419 = 1.0 ("y")
                          w425 = u8 1 items=["Channel A", "Channel B"] ("Channel A/B for Parameter1")
                          w413 = u8 0 items=["Channel A", "Channel B"] ("Channel A/B for Parameter1")
                          n82 = Format Into String(0) -> (error out=w426:errorcluster)  [unwired: 3 in, 1 out]
                          n83 = Format Into String(0) -> (error out=w415:errorcluster)  [unwired: 3 in, 1 out]
                          n84 = call "OE1022D_Read 1 parameter_mean_and_std.vi"("Num Averages"="Num Averages", "Parameter 2"="Parameter B 2", "错误输入（无错误）"=w426, "Channel (0: A)"=w425, "VISA resource name"=w412) -> ("error out"=w422:errorcluster, "Measurement"=w423:dbl, "VISA resource name out"=w421:refnum<visa-resource-name>, "Measurement STD"=w420:dbl)  [unwired: 3 in]
                          n85 = call "OE1022D_Read 1 parameter_mean_and_std.vi"("错误输入（无错误）"=w415, "Parameter"="Parameter A 2", "Channel (0: A)"=w413, "VISA resource name"=w412) -> ("error out"=w416:errorcluster, "Measurement"=w418:dbl, "VISA resource name out"=w417:refnum<visa-resource-name>, "Measurement STD"=w411:dbl)  [unwired: 4 in]
                          n86 = Multiply(x=w423, y=w419) -> (x*y=w428:dbl)
                          "para2 Measurement (uV) 2" <- w428
                          n87 = Multiply(x=w418, y=w410) -> (x*y=w427:dbl)
                          "para1 Measurement (mV) 2" <- w427
                          n88 = Multiply(x=w411, y=w410) -> (x*y=w409:dbl)
                          n89 = Build Array(w427) -> (w440:dbl[])
                          n90 = Build Array(w428) -> (w435:dbl[])
                          n91 = Select(t=w435, s="F Clear Plot B", f=w434) -> (s? t:f=w432:dbl[])
                          n92 = Select(t=w440, s="F Clear Plot A", f=w439) -> (s? t:f=w433:dbl[])
                          n93 = Build Array (concatenate)(w438, w437) -> (w429:dbl[])
                          n94 = Multiply(x=w420, y=w419) -> (x*y=w408:dbl)
                        }
                        frame #1 {
                          n95 = Wait (ms)(milliseconds to wait=u32 50) -> ()  [unwired: 1 out]
                        }
                        frame #2 {
                          n96 = Build Array (concatenate)(w505, w504) -> (w490:dbl[])
                          n97 = Build Array (concatenate)(w502, w501) -> (w489:dbl[])
                          n98 = call "OE1022D_Read 1 parameter_mean_and_std.vi"("Num Averages"=w466, "Parameter 2"="Phase B 2", "错误输入（无错误）"=w475, "Channel (0: A)"=w476, "VISA resource name"=w477) -> ("Measurement"=w479:dbl, "Measurement STD"=w468:dbl)  [unwired: 3 in, 2 out]
                          "phase B 2" <- w479
                          n99 = Bundle(w491, w490) -> (→"RA-F":cluster{dbl[], dbl[]})  [unwired: 1 in]
                          n100 = Bundle(w492, w489) -> (→"Rh1B-F":cluster{dbl[], dbl[]})  [unwired: 1 in]
                          n101 = call "OE1022D_Read 1 parameter_mean_and_std.vi"("Num Averages"=w466, "错误输入（无错误）"=w471, "Parameter"="Phase A 2", "Channel (0: A)"=w473, "VISA resource name"=w474) -> ("error out"=w470:errorcluster, "Measurement"=w469:dbl, "Measurement STD"=w467:dbl)  [unwired: 3 in, 1 out]
                          "phase A 2" <- w469
                          n102 = Divide(x=w489, y=w490) -> (x/y=w484:dbl[])
                          n103 = Build Array(w469) -> (w493:dbl[])
                          n104 = Build Array(w479) -> (w494:dbl[])
                          n105 = Select(t=w493, s=w496, f=w497) -> (s? t:f=w495:dbl[])
                          n106 = Select(t=w494, s=w499, f=w500) -> (s? t:f=w498:dbl[])
                          n107 = Sign(1:w479) -> (0:w482:dbl)
                          n108 = Negate(x=w484) -> (-x=w485:dbl[])
                          n109 = Build Array (concatenate)(w469, w495) -> (w506:dbl[])
                          n110 = Build Array (concatenate)(w479, w498) -> (w503:dbl[])
                          n111 = Greater Or Equal To 0?(x=w482) -> (x >= 0?=w483:bool)
                          n112 = Select(t=w484, s=w483, f=w485) -> (s? t:f=w486:dbl[])
                          n113 = Bundle(w508, w506) -> (→"PhaseA-F":cluster{dbl[], dbl[]})  [unwired: 1 in]
                          n114 = Bundle(w512, w503) -> (→"Phaseh1B-F":cluster{dbl[], dbl[]})  [unwired: 1 in]
                          n115 = Bundle(w488, w486) -> (→"Rh1 B/A v F":cluster{dbl[], dbl[]})  [unwired: 1 in]
                        }
                        frame #3 {
                          n116 = Wait (ms)(milliseconds to wait=u32 50) -> ()  [unwired: 1 out]
                        }
                      }
                    }
                  }
                  n117 = Build Array(w214, w216, w210, w211, w207, w212, w209, w213, w208) -> (w215:dbl[])
                  n118 = case shown="True" w220 {
                    tunnel: w217 -> [_ w244]
                    tunnel: w215 -> [_ w247]
                    frame False {
                    }
                    frame True {
                      n119 = call-poly <vilib>:"Write Delimited Spreadsheet.vi"("file path (dialog if empty)"=w244, "format (%.3f)"="%.10f", "1D data"=w247, "append to file? (new file:F)"=TRUE) -> ()  [unwired: 10 in, 2 out]
                    }
                  }
                }
              }
            }
            frame True {
              n120 = Format Into String(format string="%.0f", "Set FIxed F (Oe)") -> (resulting string=w547:string)  [unwired: 2 in, 1 out]
              n121 = Format Into String(initial string=w548, "Sweep", w545, w547, w544, w543) -> (resulting string=w549:string)  [unwired: 2 in, 1 out]
              n122 = call "SetField.vi"("Mode"="Fixed F mode", "Approach"="Fixed Field Approach", "Rate"="FIxed F Rate (Oe/s)", "Field"="Set FIxed F (Oe)", "error in (no error)"=w559, "Instrument Ref In"=w560) -> ("error out"=w555:errorcluster, "Instrument Ref Out"=w557:refnum<k24>)  [unwired: 1 in, 1 out]
              n123 = Build Array(" #T(Oe) R(V) theta(deg) dR(V) dRtheta(deg)") -> (w536:string[])
              n124 = call "WaitFor.vi"("Delay"=w553, "Wait For Field"=TRUE, "error in (no error)"=w555, "Instrument Ref In"=w557) -> ("error out"=w556:errorcluster, "Instrument Ref Out"=w558:refnum<k24>)  [unwired: 6 in]
              n125 = String To Path(string=w549) -> (path=w533:path)
              n126 = call-poly <vilib>:"Write Delimited Spreadsheet.vi"("file path (dialog if empty)"=w533, "1D data"=w536, "append to file? (new file:F)"=TRUE) -> ("new file path (Not A Path if cancelled)"=w532:path)  [unwired: 11 in, 1 out]
              n127 = for {
                N: w564 -> [_]
                tunnel: w565 -> [w595]
                tunnel: "Low Value (K)" -> [w589]
                tunnel: "High Value (K)" -> [w579]
                tunnel: w532 -> [w588]
                shift-right: [w584] -> _
                shift-left: _ -> [w583]
                shift-right: [w578] -> _
                shift-left: _ -> [w577]
                shift-right: [w576] -> _
                shift-left: _ -> [w575]
                shift-right: [w574] -> _
                shift-left: _ -> [w573]
                tunnel: w558 -> [w572]
                tunnel: w556 -> [w571]
                tunnel: w552 -> [w570]
                tunnel: w540 -> [w569]
                tunnel: [w568] -> w539
                tunnel: [w567] -> w538
                tunnel: w537 -> [w566]
                i -> [w581]
                n128 = Subtract(x=w579, y=w589) -> (x-y=w591:dbl)
                n129 = Add(x=1, y=w581) -> (x+y=→"T loop run":i32)
                n130 = Divide(x="Step(K)", y=1) -> (x/y=w590:dbl)
                n131 = Divide(x=w591, y=w590) -> (x/y=w587:dbl)
                n132 = Multiply(x=2, y=w587) -> (x*y=w586:dbl)
                n133 = Increment(x=w586) -> (x+1=w585:dbl)
                n134 = for {
                  N: w585 -> [_]
                  tunnel: w595 -> [w627]
                  tunnel: w590 -> [w623]
                  shift-right: [w614] -> w584
                  shift-left: w583 -> [w626]
                  tunnel: w587 -> [w621]
                  tunnel: w589 -> [w624]
                  tunnel: w579 -> [w622]
                  tunnel: w588 -> [w598]
                  shift-right: [w603] -> _
                  shift-left: _ -> [w617]
                  shift-right: [w616] -> w578
                  shift-left: w577 -> [w615]
                  shift-right: [w613] -> w576
                  shift-left: w575 -> [w612]
                  shift-right: [w611] -> w574
                  shift-left: w573 -> [w610]
                  tunnel: w572 -> [w609]
                  tunnel: w571 -> [w608]
                  tunnel: w570 -> [w607]
                  tunnel: w569 -> [w606]
                  tunnel: [w605] -> w568
                  tunnel: [w604] -> w567
                  tunnel: w566 -> [w596]
                  i -> [w620]
                  n135 = Less Or Equal?(x=w620, y=w621) -> (x <= y?=w625:bool)
                  n136 = case shown="False" w625 {
                    tunnel: w624 -> [w637 w665]
                    tunnel: w620 -> [w646 w664]
                    tunnel: w623 -> [w645 w663]
                    tunnel: [w643 w661] -> w619
                    tunnel: w622 -> [w644 _]
                    tunnel: w621 -> [w639 _]
                    tunnel: w620 -> [w642 _]
                    frame False {
                      n137 = Multiply(x=w639, y=2) -> (x*y=w638:dbl)
                      n138 = Less Or Equal?(x=w642, y=w638) -> (x <= y?=w640:bool)
                      n139 = case shown="False" w640 {
                        tunnel: w646 -> [w653 w660]
                        tunnel: w645 -> [w651 w658]
                        tunnel: w644 -> [_ w656]
                        tunnel: [w649 w655] -> w643
                        tunnel: w639 -> [_ w654]
                        tunnel: w638 -> [w648 _]
                        tunnel: w637 -> [w647 _]
                        frame False {
                          n140 = Subtract(x=w653, y=w648) -> (x-y=w652:dbl)
                          n141 = Multiply(x=w651, y=w652) -> (x*y=w650:dbl)
                          n142 = Add(x=w647, y=w650) -> (x+y=w649:dbl)
                        }
                        frame True {
                          n143 = Subtract(x=w660, y=w654) -> (x-y=w659:dbl)
                          n144 = Multiply(x=w658, y=w659) -> (x*y=w657:dbl)
                          n145 = Subtract(x=w656, y=w657) -> (x-y=w655:dbl)
                        }
                      }
                    }
                    frame True {
                      n146 = Multiply(x=w663, y=w664) -> (x*y=w662:dbl)
                      n147 = Add(x=w665, y=w662) -> (x+y=w661:dbl)
                    }
                  }
                  n148 = Absolute Value(x=w619) -> (abs(x)=w618:dbl)
                  n149 = stacked-sequence {
                    tunnel: w627 -> [_ _ w766]
                    tunnel: w618 -> [w684 _ w704]
                    tunnel: w626 -> [_ _ w768]
                    tunnel: [_ _ w767] -> w614
                    tunnel: [_ _ w765] -> w599
                    tunnel: [_ _ w764] -> w603
                    tunnel: w617 -> [_ _ w763]
                    tunnel: [_ _ w762] -> w600
                    tunnel: [_ _ w761] -> w616
                    tunnel: w615 -> [_ _ w755]
                    tunnel: [_ _ w760] -> w613
                    tunnel: w612 -> [_ _ w756]
                    tunnel: [_ _ w759] -> w611
                    tunnel: w610 -> [_ _ w758]
                    tunnel: [_ _ w705] -> w601
                    tunnel: [_ _ w757] -> w602
                    tunnel: w609 -> [w683 _ _]
                    tunnel: w608 -> [w682 _ _]
                    tunnel: w607 -> [w679 _ _]
                    tunnel: w606 -> [_ w701 _]
                    tunnel: [w667 _ _] -> w605
                    tunnel: [w666 _ _] -> w604
                    tunnel: [_ _ w704] -> w597
                    frame #0 {
                      n150 = call "SetTemperature.vi"("Approach"="Sweep Temperature Approach", "Rate"="Sweep T  Rate (K/min)", "Temperature"=w684, "error in (no error)"=w682, "Instrument Ref In"=w683) -> ("error out"=w680:errorcluster, "Instrument Ref Out"=w681:refnum<k24>)  [unwired: 2 in, 1 out]
                      n151 = call "WaitFor.vi"("Delay"=w679, "Wait For Temperature"=TRUE ("WaitForTemperature"), "error in (no error)"=w680, "Instrument Ref In"=w681) -> ("error out"=w670:errorcluster, "Instrument Ref Out"=w669:refnum<k24>)  [unwired: 6 in]
                      n152 = for {
                        N: 20 -> [_]
                        shift-right: [w700] -> _
                        shift-left: TRUE -> [w698]
                        shift-right: [w695] -> w667
                        shift-left: w670 -> [w697]
                        tunnel: w669 -> [w694]
                        tunnel: [w692] -> w666
                        tunnel: [w689] -> w676
                        tunnel: [w688] -> w675
                        tunnel: [w690] -> w673 mode=indexing
                        tunnel: [w691] -> w674 mode=indexing
                        n153 = local write "Measuring T"(w698) -> ()
                        n154 = Not(x=w698) -> (.not. x?=w700:bool)
                        n155 = call "GetTemperature.vi"("error in (no error)"=w697, "Instrument Ref In"=w694) -> ("Temperature\nStatus"=w688:i32, "Temperature"=w691:dbl, "error out"=w696:errorcluster, "Instrument Ref Out"=w693:refnum<k24>)  [unwired: 3 in, 1 out]
                        n156 = Wait (ms)(milliseconds to wait=u32 200) -> ()  [unwired: 1 out]
                        n157 = call "GetField.vi"("error in (no error)"=w696, "Instrument Ref In"=w693) -> ("Field\nStatus"=w689:i32, "Field"=w690:dbl, "error out"=w695:errorcluster, "Instrument Ref Out"=w692:refnum<k24>)  [unwired: 3 in, 1 out]
                      }
                      "Field Status" <- w676
                      "Temperature Status" <- w675
                      n158 = call-poly <vilib>:"Mean.vi"("X"=w673) -> ("mean"=→"Fixed Field":dbl)  [unwired: 1 out]
                      n159 = call-poly <vilib>:"Mean.vi"("X"=w674) -> ("mean"=→"Measured Temperature":dbl)  [unwired: 1 out]
                      "Temperature Setting" <- w684
                      "Measuring T" <- FALSE
                    }
                    frame #1 {
                      n160 = Multiply(x=w701, y=1000) -> (x*y=w703:dbl)
                      n161 = Wait (ms)(milliseconds to wait=w703) -> ()  [unwired: 1 out]
                    }
                    frame #2 {
                      n162 = flat-sequence {
                        tunnel: w768 -> [w796]
                        tunnel: w766 -> [w787]
                        tunnel: w704 -> [w795]
                        tunnel: w763 -> [w794]
                        tunnel: w758 -> [w785]
                        tunnel: [w792] -> w754
                        tunnel: [w779] -> w752
                        tunnel: [w780] -> w750
                        tunnel: [w777] -> w748
                        tunnel: [w780] -> w746
                        tunnel: [w780] -> w744
                        tunnel: [w780] -> w742
                        tunnel: [w780] -> w740
                        tunnel: [w779] -> w738
                        tunnel: [w778] -> w736
                        tunnel: [w777] -> w734
                        tunnel: [w776] -> w732
                        tunnel: ["T Clear Plot B"] -> w730
                        tunnel: ["T Clear Plot A"] -> w728
                        tunnel: [w773] -> w726
                        tunnel: [w772] -> w724
                        tunnel: [w771] -> w722
                        tunnel: [w770] -> w720
                        tunnel: [w769] -> w718
                        tunnel: w754 -> [w818]
                        tunnel: [w818] -> w753
                        tunnel: w752 -> [w817]
                        tunnel: [w817] -> w751
                        tunnel: w750 -> [w816]
                        tunnel: [w816] -> w749
                        tunnel: w748 -> [w815]
                        tunnel: [w815] -> w747
                        tunnel: w746 -> [w814]
                        tunnel: [w814] -> w745
                        tunnel: w744 -> [w813]
                        tunnel: [w813] -> w743
                        tunnel: w742 -> [w812]
                        tunnel: [w812] -> w741
                        tunnel: w740 -> [w811]
                        tunnel: [w811] -> w739
                        tunnel: w738 -> [w810]
                        tunnel: [w810] -> w737
                        tunnel: w736 -> [w809]
                        tunnel: [w809] -> w735
                        tunnel: w734 -> [w808]
                        tunnel: [w808] -> w733
                        tunnel: w732 -> [w807]
                        tunnel: [w807] -> w731
                        tunnel: w730 -> [w806]
                        tunnel: [w806] -> w729
                        tunnel: w728 -> [w805]
                        tunnel: [w805] -> w727
                        tunnel: w726 -> [w804]
                        tunnel: [w804] -> w725
                        tunnel: w724 -> [w803]
                        tunnel: [w803] -> w723
                        tunnel: w722 -> [w802]
                        tunnel: [w802] -> w721
                        tunnel: w720 -> [w801]
                        tunnel: [w801] -> w719
                        tunnel: w718 -> [w800]
                        tunnel: [w800] -> w717
                        tunnel: w753 -> [w822]
                        tunnel: w751 -> [w856]
                        tunnel: w749 -> [w855]
                        tunnel: w747 -> [w854]
                        tunnel: w745 -> [w853]
                        tunnel: w743 -> [w851]
                        tunnel: w741 -> [w849]
                        tunnel: w739 -> [w847]
                        tunnel: w737 -> [w844]
                        tunnel: w735 -> [w843]
                        tunnel: w733 -> [w840]
                        tunnel: w731 -> [w839]
                        tunnel: w756 -> [w837]
                        tunnel: w729 -> [w836]
                        tunnel: w755 -> [w834]
                        tunnel: w727 -> [w833]
                        tunnel: w725 -> [w829]
                        tunnel: w723 -> [w828]
                        tunnel: w721 -> [w827]
                        tunnel: w719 -> [w824]
                        tunnel: w717 -> [w823]
                        tunnel: [w822] -> w716
                        tunnel: [w842] -> w715
                        tunnel: [w856] -> w714
                        tunnel: [w855] -> w713
                        tunnel: [w820] -> w712
                        tunnel: [w821] -> w711
                        tunnel: [w845] -> w710
                        tunnel: [w841] -> w709
                        tunnel: [w838] -> w708
                        tunnel: [w854] -> w707
                        tunnel: [w826] -> w706
                        tunnel: [w860] -> w757
                        tunnel: [w861] -> w705
                        tunnel: [w858] -> w759
                        tunnel: [w862] -> w760
                        tunnel: [w863] -> w761
                        tunnel: [w864] -> _
                        tunnel: [w865] -> w762
                        tunnel: [w866] -> w764
                        tunnel: [w867] -> w765
                        tunnel: [w857] -> w767
                        tunnel: [w868] -> _
                        tunnel: w716 -> [w868]
                        tunnel: w715 -> [w857]
                        tunnel: w714 -> [w867]
                        tunnel: w713 -> [w866]
                        tunnel: w712 -> [w865]
                        tunnel: w711 -> [w864]
                        tunnel: w710 -> [w863]
                        tunnel: w709 -> [w862]
                        tunnel: w708 -> [w858]
                        tunnel: w707 -> [w861]
                        tunnel: w706 -> [w860]
                        frame #0 {
                          w772 = u8 1 items=["Channel A", "Channel B"] ("Channel A/B for Parameter1")
                          w769 = u8 0 items=["Channel A", "Channel B"] ("Channel A/B for Parameter1")
                          n163 = Format Into String(0) -> (error out=w793:errorcluster)  [unwired: 3 in, 1 out]
                          n164 = Format Into String(0) -> (error out=w788:errorcluster)  [unwired: 3 in, 1 out]
                          n165 = call "OE1022D_Read 1 parameter_mean_and_std.vi"("错误输入（无错误）"=w793, "Parameter"="Parameter A", "Channel (0: A)"=w769, "VISA resource name"=w787) -> ("error out"=w770:errorcluster, "Measurement"=w782:dbl, "VISA resource name out"=w792:refnum<visa-resource-name>)  [unwired: 4 in, 1 out]
                          n166 = call "OE1022D_Read 1 parameter_mean_and_std.vi"("Parameter 2"="Parameter B", "错误输入（无错误）"=w788, "Channel (0: A)"=w772, "VISA resource name"=w787) -> ("error out"=w773:errorcluster, "Measurement"=w781:dbl, "VISA resource name out"=w771:refnum<visa-resource-name>)  [unwired: 4 in, 1 out]
                          n167 = Multiply(x=w782, y=1000.0) -> (x*y=w779:dbl)
                          "para1 Measurement (mV)" <- w779
                          n168 = Multiply(x=w781, y=1000000.0) -> (x*y=w777:dbl)
                          "para2 Measurement (uV)" <- w777
                          n169 = Build Array(w779) -> (w797:dbl[])
                          n170 = Build Array(w777) -> (w789:dbl[])
                          n171 = Select(t=w797, s="T Clear Plot A", f=w796) -> (s? t:f=w778:dbl[])
                          n172 = Select(t=w789, s="T Clear Plot B", f=w785) -> (s? t:f=w776:dbl[])
                          n173 = Build Array (concatenate)(w795, w794) -> (w780:dbl[])
                        }
                        frame #1 {
                          n174 = Wait (ms)(milliseconds to wait=u32 50) -> ()  [unwired: 1 out]
                        }
                        frame #2 {
                          n175 = Build Array (concatenate)(w844, w843) -> (w842:dbl[])
                          n176 = Build Array (concatenate)(w840, w839) -> (w838:dbl[])
                          n177 = Bundle(w849, w842) -> (→"RA-T":cluster{dbl[], dbl[]})  [unwired: 1 in]
                          n178 = Bundle(w851, w838) -> (→"Rh1B-T":cluster{dbl[], dbl[]})  [unwired: 1 in]
                          n179 = call "OE1022D_Read 1 parameter_mean_and_std.vi"("错误输入（无错误）"=w824, "Parameter"="Phase A", "Channel (0: A)"=w823, "VISA resource name"=w822) -> ("error out"=w821:errorcluster, "Measurement"=w820:dbl)  [unwired: 4 in, 2 out]
                          "phase A" <- w820
                          n180 = call "OE1022D_Read 1 parameter_mean_and_std.vi"("Parameter 2"="Phase B", "错误输入（无错误）"=w829, "Channel (0: A)"=w828, "VISA resource name"=w827) -> ("Measurement"=w826:dbl)  [unwired: 4 in, 3 out]
                          "phase B" <- w826
                          n181 = Build Array(w820) -> (w830:dbl[])
                          n182 = Build Array(w826) -> (w831:dbl[])
                          n183 = Select(t=w830, s=w833, f=w834) -> (s? t:f=w832:dbl[])
                          n184 = Select(t=w831, s=w836, f=w837) -> (s? t:f=w835:dbl[])
                          n185 = Build Array (concatenate)(w820, w832) -> (w845:dbl[])
                          n186 = Build Array (concatenate)(w826, w835) -> (w841:dbl[])
                          n187 = Bundle(w847, w845) -> (→"PhaseA-T":cluster{dbl[], dbl[]})  [unwired: 1 in]
                          n188 = Bundle(w853, w841) -> (→"Phaseh1-T":cluster{dbl[], dbl[]})  [unwired: 1 in]
                        }
                        frame #3 {
                          n189 = Wait (ms)(milliseconds to wait=u32 50) -> ()  [unwired: 1 out]
                        }
                      }
                    }
                  }
                  n190 = case shown="True" w596 {
                    tunnel: w599 -> [_ w631]
                    tunnel: w597 -> [_ w636]
                    tunnel: w598 -> [_ w634]
                    tunnel: w600 -> [_ w630]
                    tunnel: w601 -> [_ w629]
                    tunnel: w602 -> [_ w628]
                    frame False {
                    }
                    frame True {
                      n191 = Build Array(w636, w631, w630, w629, w628) -> (w633:dbl[])
                      n192 = call-poly <vilib>:"Write Delimited Spreadsheet.vi"("file path (dialog if empty)"=w634, "format (%.3f)"="%.10f", "1D data"=w633, "append to file? (new file:F)"=TRUE) -> ()  [unwired: 10 in, 2 out]
                    }
                  }
                }
              }
            }
          }
        }
      }
    }
    frame #2 {
      n193 = case shown="False" "Initialize" {
        tunnel: w871 -> [w872 w875]
        tunnel: w870 -> [w873 w874]
        frame False {
          n194 = Close Reference(reference=w873, error in (no error)=w872) -> ()  [unwired: 1 out]
        }
        frame True {
          w881 = 0 items=["Linear", "NoOvershoot", "Oscillate"] ("Approach")
          w882 = 0 items=["Persistent", "Driven"] ("Mode")
          w878 = 0 items=["FastSettle", "NoOvershoot"] ("Approach")
          n195 = call "SetTemperature.vi"("Approach"=w878, "Rate"=20.0, "Temperature"=2.0, "error in (no error)"=w875, "Instrument Ref In"=w874) -> ("error out"=w886:errorcluster, "Instrument Ref Out"=w885:refnum<k24>)  [unwired: 2 in, 1 out]
          n196 = call "SetField.vi"("Mode"=w882, "Approach"=w881, "Rate"=200.0, "Field"=0.0, "error in (no error)"=w886, "Instrument Ref In"=w885) -> ("error out"=w883:errorcluster, "Instrument Ref Out"=w884:refnum<k24>)  [unwired: 1 in, 1 out]
          n197 = Close Reference(reference=w884, error in (no error)=w883) -> ()  [unwired: 1 out]
        }
      }
    }
    frame #3 {
    }
  }
  n198 = case shown="True" "Read Status" {
    tunnel: w5 -> [_ w890]
    tunnel: w4 -> [_ w889]
    tunnel: w2 -> [_ w888]
    frame False {
    }
    frame True {
      n199 = while {
        tunnel: w890 -> [w893]
        tunnel: w889 -> [w892]
        tunnel: w888 -> [w891]
        stop <- w891 stop-if-true
        n200 = for {
          N: 10 -> [_]
          shift-right: [w908] -> _
          shift-left: w892 -> [w910]
          tunnel: w893 -> [w907]
          tunnel: [w905] -> _
          tunnel: [w902] -> w899
          tunnel: [w901] -> w898
          tunnel: [w903] -> w896 mode=indexing
          tunnel: [w904] -> w897 mode=indexing
          n201 = call "GetTemperature.vi"("error in (no error)"=w910, "Instrument Ref In"=w907) -> ("Temperature\nStatus"=w901:i32, "Temperature"=w904:dbl, "error out"=w909:errorcluster, "Instrument Ref Out"=w906:refnum<k24>)  [unwired: 3 in, 1 out]
          n202 = Wait (ms)(milliseconds to wait=u32 200) -> ()  [unwired: 1 out]
          n203 = call "GetField.vi"("error in (no error)"=w909, "Instrument Ref In"=w906) -> ("Field\nStatus"=w902:i32, "Field"=w903:dbl, "error out"=w908:errorcluster, "Instrument Ref Out"=w905:refnum<k24>)  [unwired: 3 in, 1 out]
        }
        "Field Status" <- w899
        "Temperature Status" <- w898
        n204 = call-poly <vilib>:"Mean.vi"("X"=w896) -> ("mean"=→"Field":dbl)  [unwired: 1 out]
        n205 = call-poly <vilib>:"Mean.vi"("X"=w897) -> ("mean"=→"Temperature":dbl)  [unwired: 1 out]
      }
    }
  }
